vi "Write Last error.vi"(8 "error in (no error)":errorcluster, 10 "Last error":errorcluster, 11 "RP Communicator in":refnum<class "RP Communicator.lvclass">) -> (0 "error out":errorcluster, 3 "RP Communicator out":refnum<class "RP Communicator.lvclass">)   [LabVIEW 2021, in "RP Communicator.lvclass"]
uses:
  RP Communicator.lvclass
  RP Communicator.lvclass/RP Communicator.ctl
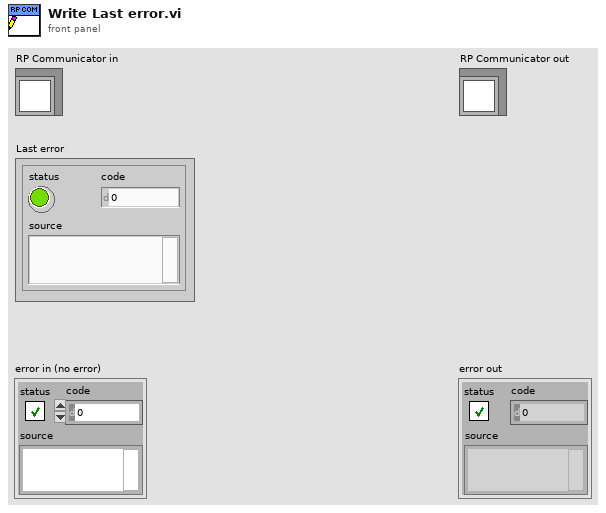
[diagram p1: front panel]
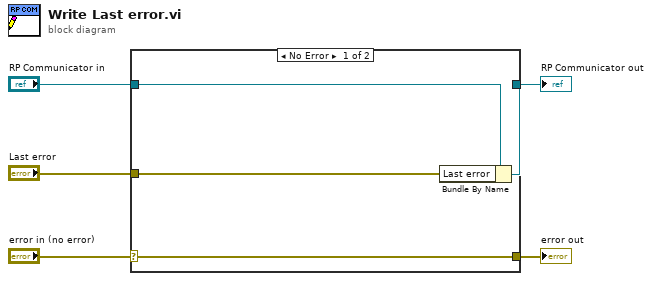
[diagram p0: block diagram]
diagram:
  n1 = case shown="No Error" "error in (no error)" {
    selector: "error in (no error)" -> [w9 w10]
    tunnel: [w9 w10] -> w4
    tunnel: [w7 w11] -> w2
    tunnel: "RP Communicator in" -> [w8 w11]
    tunnel: "Last error" -> [w6 _]
    frame No Error {
      n2 = Bundle By Name(cluster=w8, "Last error"=w6) -> (w7:refnum<class "RP Communicator.lvclass">)
    }
    frame Error {
    }
  }
  "error out" <- w4
  "RP Communicator out" <- w2
